vi "Change_Beam_Check_Positions.vi"   [LabVIEW 2011]
types:
  T1 = enum16{"Load setup from excel file", "Save setup to excel file"}
  T2 = enum16{"Load From Excel File", "Save to Excel File"}
  T3 = typedef "LDA_Beam_Cluster.ctl" = cluster{"Vg1 (Green 1 dir. vect.)":dbl[], "Vg2  (Green 2 dir. vect.)":dbl[], "Vb1 (Blue 1 dir. vect.)":dbl[], "Vb2 (Blue 1 dir. vect.)":dbl[], "Porb (Orb XYZ posn. forced coplanar)":dbl[], "Porb (Orb XYZ posn. - allow skew)":dbl[], "Orb posn. uncertainty, +/- dx, dy, dz":dbl[], "Vp (Actual Probe dir. vect)":dbl[], "Yaw (deg)":dbl, "Pitch (deg)":dbl, "In-Plane Roll (deg)":dbl, "Beam Half Angle (deg)":dbl, "B1 Close P11":dbl[], "B1 Far P12":dbl[], "B2 Close P22":dbl[], "B2 Far P21":dbl[], "Projected Roll (deg)":dbl, "Green Velocity Vector":dbl[], "Blue Velocity Vector":dbl[], "Probe is facing....":string, "Calculation Method":string}
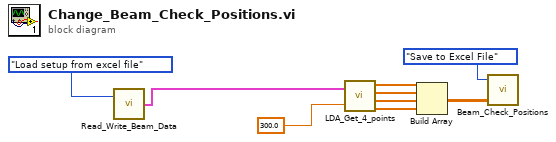
[diagram p0: block diagram]
diagram:
  n1 = call "Read_Write_Beam_Data.vi"("Mode"=T1."Load setup from excel file") -> ("Beam Data Out"=w7:T3)  [unwired: 1 in]
  n2 = call "LDA_Get_4_points.vi"("Beam Data"=w7, "L, Probe-Normal Distance"=300.0) -> ("Pg1"=w5:dbl[], "Pg2"=w4:dbl[], "Pb1"=w3:dbl[], "Pb2"=w2:dbl[])
  n3 = Build Array(w5, w4, w3, w2) -> (w1:dbl[][])
  n4 = call "Beam_Check_Positions.vi"("Values"=w1, "Mode"=T2."Save to Excel File") -> ()  [unwired: 2 out]
